vi "SUB InstantPhase_v3.vi"(10 "Unwrap":bool, 11 "Waveform":waveform(dbl)) -> (3 "Instantaneous Phase":waveform(dbl))   [LabVIEW 2017]
uses:
  <vilib>/Analysis/NI_AALPro.lvlib
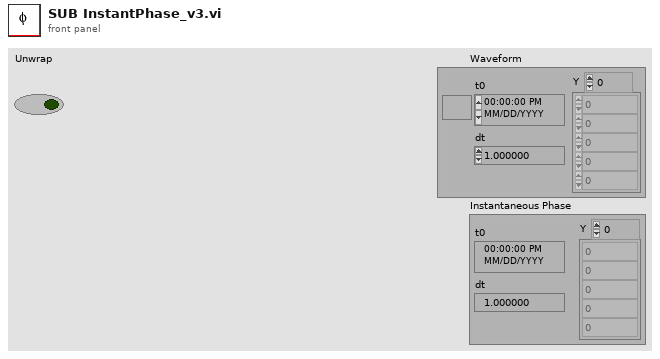
[diagram p1: front panel]
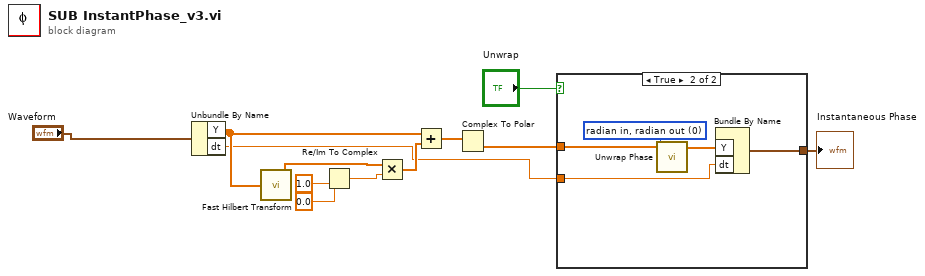
[diagram p0: block diagram]
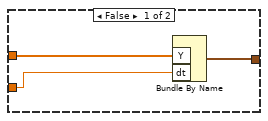
[diagram p2: hidden frame]
diagram:
  n1 = Unbundle By Name("Waveform") -> ("Y"=w7:dbl[], "dt"=w3:dbl)
  n2 = call <vilib>:"Fast Hilbert Transform.vi"("X"=w7) -> ("Hilbert{X}"=w10:dbl[])  [unwired: 1 out]
  n3 = Re/Im To Complex(1:1.0 ("y"), 2:0.0 ("x")) -> (0:w11:cdb)
  n4 = Multiply(x=w10, y=w11) -> (x*y=w9:cdb[])
  n5 = Add(x=w7, y=w9) -> (x+y=w8:cdb[])
  n6 = Complex To Polar(r * e^(i*theta)=w8) -> (theta=w4:dbl[])  [unwired: 1 out]
  n7 = case shown="True" "Unwrap" {
    tunnel: w4 -> [w15 w18]
    tunnel: w3 -> [w14 w17]
    tunnel: [w13 w16] -> w2
    frame False {
      n8 = Bundle By Name("Y"=w15, "dt"=w14) -> (w13:waveform(dbl))  [unwired: 1 in]
    }
    frame True {
      w20 = 0 items=["radian in, radian out", "radian in, degree out", "degree in, degree out", "degree in, radian out"] ("phase unit")
      n9 = call <vilib>:"Unwrap Phase.vi"("phase unit"=w20, "Phase"=w18) -> ("Unwrapped Phase"=w19:dbl[])  [unwired: 8 in, 1 out]
      n10 = Bundle By Name("Y"=w19, "dt"=w17) -> (w16:waveform(dbl))  [unwired: 1 in]
    }
  }
  "Instantaneous Phase" <- w2
